vi "ASM.Doom.vi"(8 "error in (no error)":errorcluster, 11 "AsmTestMachine in":refnum<class "AsmTestMachine.lvclass">) -> (0 "error out":errorcluster, 3 "AsmTestMachine out":refnum<class "AsmTestMachine.lvclass">)   [LabVIEW 2021, in "AsmTestMachine.lvlib" / "AsmTestMachine.lvclass"]
uses:
  AsmTestMachine.lvclass
  AsmTestMachine.lvclass/AsmTestMachine.ctl
  Source/ActorStateMachine/ActorStateMachine/ActorStateMachine.lvclass
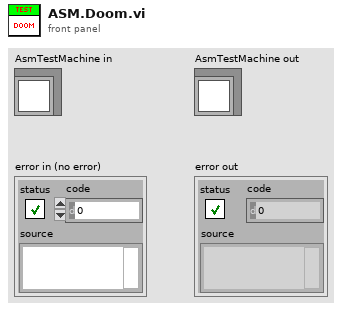
[diagram p1: front panel]
types:
  T1 = enum32{"Invalid", "Standard", "Closed", "Hidden", "Minimized", "Maximized"}
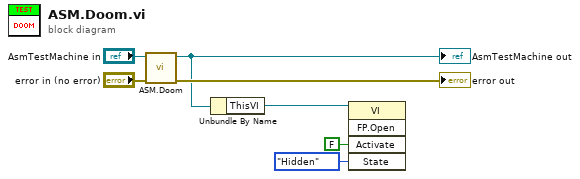
[diagram p0: block diagram]
diagram:
  n1 = call-parent "ASM.Doom.vi"("error in (no error)"="error in (no error)", "ActorStateMachine in"="AsmTestMachine in") -> ("error out"=→"error out":errorcluster, "ActorStateMachine out"=w4:refnum<class "AsmTestMachine.lvclass">)  [unwired: 8 in]
  "AsmTestMachine out" <- w4
  n2 = Unbundle By Name(w4) -> ("ThisVI"=w1:refnum<vi>)
  n3 = invoke class="VI" method="FP.Open"(reference=w1, "Activate"=FALSE ("Activate?"), "State"=T1."Hidden") -> ()  [unwired: 2 in, 5 out]
